vi "z reply err clone.vi"(8 "error in (no error)":errorcluster, 10 "this_":cluster{}, 11 "dst":cluster{}) -> (0 "error out":errorcluster, 3 "dst out":cluster{})   [LabVIEW 2021, in "zenohc.lvlib"]
doc: "void z_reply_err_clone(struct z_owned_reply_err_t *dst,\n const struct z_loaned_reply_err_t *this_);"
uses:
  zenohc.lvlib
  zenohc.dll
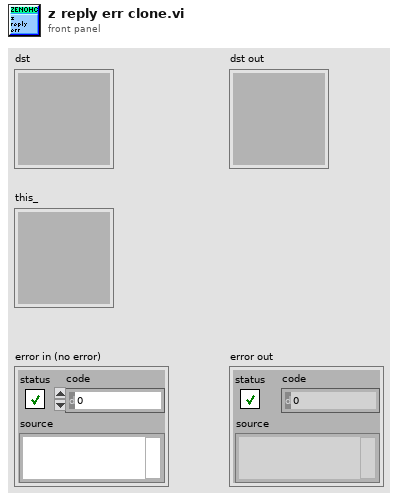
[diagram p1: front panel]
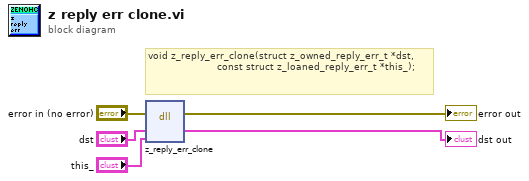
[diagram p0: block diagram]
diagram:
  # "void z_reply_err_clone(struct z_owned_reply_err_t *dst,\n                       const struct z_loaned_reply_err_t *this_);"
  n1 = dll-call lib="D:/dev/zenoh_labview/zenohc/zenohc.*" fn="z_reply_err_clone"(error in="error in (no error)", "dst"="dst", "this_"="this_") -> (error out=→"error out":errorcluster, "dst"=→"dst out":cluster{})  [unwired: 4 in, 1 out]
